vi "Gather Mean.vi"(10 "JSON Value":refnum<class "JSON Value.lvclass">, 11 "Statistics in":refnum<class "JSON Value.lvclass">) -> (3 "Statistics out":refnum<class "JSON Value.lvclass">)   [LabVIEW 2020, in "Library Commun.lvlib" / "JSON Value.lvclass"]
uses:
  JSON Value.lvclass
  JSON Running Mean/JSON Running Mean.lvclass
  C:/Users/ngarcin/OneDrive - Altyor/Standard TB/Class/JSON API/JSON Value/JSON Value.lvclass
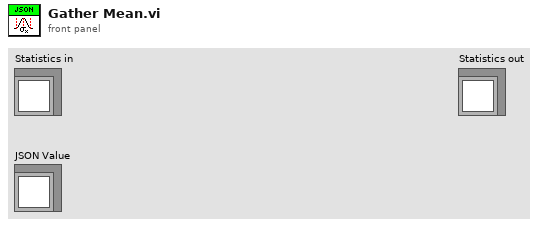
[diagram p1: front panel]
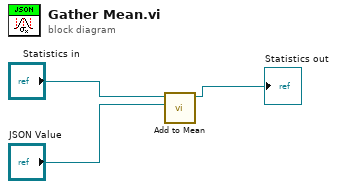
[diagram p0: block diagram]
diagram:
  n1 = call-dynamic "Add to Mean.vi"("Non Object"="JSON Value", "JSON Value In"="Statistics in") -> ("JSON Mean out"=→"Statistics out":refnum<class "JSON Running Mean.lvclass">)  [unwired: 9 in]
